vi "dcimgToTif.vi"(0 "tifPath":path, 1 "dcimgPath":path) -> ()   [LabVIEW 2015]
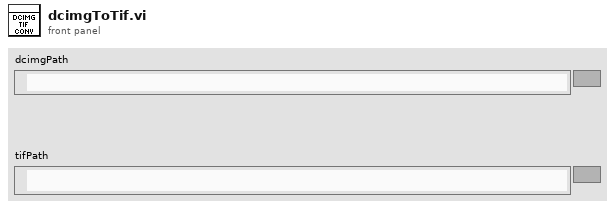
[diagram p1: front panel]
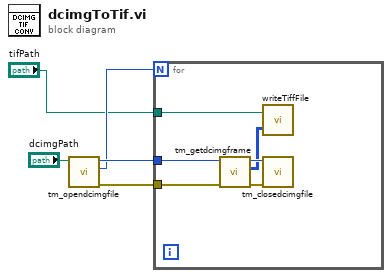
[diagram p0: block diagram]
diagram:
  n1 = call <userlib>:"tm_opendcimgfile.vi"("Path"="dcimgPath") -> ("error out"=w3:errorcluster, "Total Frames"=w2:i32, "File Handle"=w5:u32)  [unwired: 8 in]
  n2 = for {
    N: w2 -> [_]
    tunnel: w5 -> [w9]
    tunnel: w3 -> [w8]
    tunnel: "tifPath" -> [w6]
    n3 = call <userlib>:"tm_getdcimgframe.vi"("error in (no error)"=w8, "File Handle in"=w9) -> ("error out"=w7:errorcluster, "Data"=w10:u16[][], "File Handle out"=w11:u32)  [unwired: 6 in, 1 out]
    n4 = call "writeTiffFile.vi"("Image Pixels (U16)"=w10, "File Path"=w6) -> ()
    n5 = call <userlib>:"tm_closedcimgfile.vi"("error in (no error)"=w7, "File Handle"=w11) -> ()  [unwired: 9 in, 1 out]
  }
